vi "Write Cycle Time.vi"(8 "error in (no error)":errorcluster, 10 "Cyle (ms)":i32, 11 "FHPP in":refnum<class "FHPP.lvclass">) -> (0 "error out":errorcluster, 3 "FHPP out":refnum<class "FHPP.lvclass">)   [LabVIEW 2022 SP3, in "FHPP.lvclass"]
uses:
  FHPP.lvclass
  FHPP.lvclass/FHPP.ctl
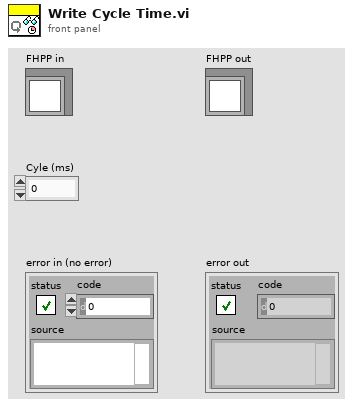
[diagram p1: front panel]
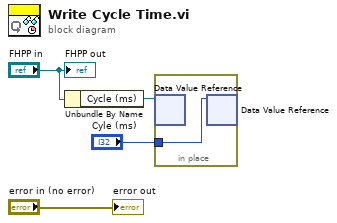
[diagram p0: block diagram]
diagram:
  n1 = Unbundle By Name("FHPP in") -> ("Cycle (ms)"=w1:refnum<data-value>)
  n2 = in-place {
    in-place-border: "Cyle (ms)" -> [w5]
    n3 = in-place-dvr #1(w1) -> ()  [unwired: 2 out]
    n4 = in-place-dvr #1(w5) -> ()  [unwired: 2 out]
  }
  "error out" <- "error in (no error)"
  "FHPP out" <- "FHPP in"
